vi "Test Recieved File Generation When Test Fails.vi"(11 "Test Case In":refnum<class "Basic Mechanics Tests.lvclass">) -> (0 "error out":errorcluster, 3 "Test Case Out":refnum<class "Basic Mechanics Tests.lvclass">)   [LabVIEW 2020, in "Basic Mechanics Tests.lvclass"]
uses:
  Basic Mechanics Tests.lvclass
  C:/Program Files/National Instruments/LabVIEW 2025/vi.lib/Astemes/LUnit/Test Case.lvclass
  Source/Approval Tests/Options/Options.lvclass
  Source/Approval Tests/Report Nothing/Report Nothing.lvclass
  C:/Users/SAS/Desktop/ApprovalTests.LabVIEW/Source/Approval Tests/Reporter/Reporter.lvclass
  Source/Approval Tests/Options/Options.lvclass/Options.ctl
  Source/Approval Tests/Naming Data/Naming Data.lvclass/Naming Data.ctl
  <vilib>/Astemes/LUnit/Test Case.lvclass/Test Case.ctl
  Source/Approval Tests/Scrubber/Scrubber.lvclass
  Source/Approval Tests/Namer/Namer.lvclass
  Source/Approval Tests/Naming Data/Naming Data.lvclass
  Source/Approval Tests/Reporter/Reporter.lvclass
  Source/Approval Tests/Text Comparator/Text Comparator.lvclass
  Basic Mechanics Tests.lvclass/Basic Mechanics Tests.ctl
  4be351cf-9afa-44a9-9686-c31d6937e1da.vi
  <vilib>/Astemes/LUnit/Test Case.lvclass
  5b6af433-73f2-478c-ac60-49e9a84e5db2.vi
  fbf3a6f1-25d3-4b1a-9ed1-fe282719be7b.vi
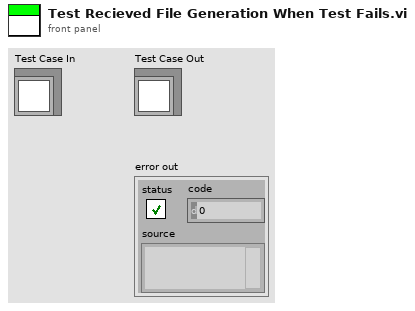
[diagram p1: front panel]
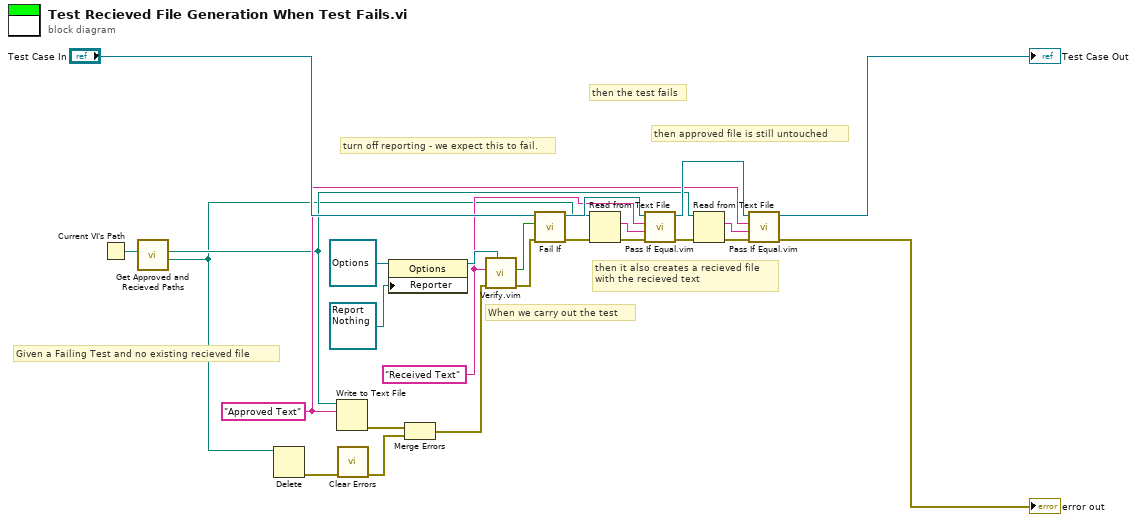
[diagram p0: block diagram]
diagram:
  w5 = "Approved Text"
  w9 = "Received Text"
  # "then approved file is still untouched"
  # "then it also creates a recieved file\nwith the recieved text"
  # "then the test fails"
  # "When we carry out the test"
  # "Given a Failing Test and no existing recieved file"
  # "turn off reporting - we expect this to fail."
  n1 = Current VI's Path() -> (path=w3:path)
  n2 = call "Get Approved and Recieved Paths.vi"("This VI"=w3) -> ("Recieved"=w1:path, "Approved Path"=w2:path)  [unwired: 9 in]
  n3 = Delete(path (use dialog)=w1) -> (error out=w25:errorcluster)  [unwired: 4 in, 2 out]
  n4 = Write to Text File(file (use dialog)=w2, text=w5) -> (error out=w24:errorcluster)  [unwired: 2 in, 2 out]
  n5 = call <vilib>:"Clear Errors.vi"("error in (no error)"=w25) -> ("error out"=w23:errorcluster)  [unwired: 5 in, 1 out]
  n6 = property on="Property Node" class="Options"(reference=refnum<class "Options.lvclass"> refnum ("Options"), "Reporter"=refnum<class "Report Nothing.lvclass"> refnum ("Approval Tests.lvlib:Report Nothing")) -> (reference out=w13:refnum<class "Options.lvclass">)  [unwired: 1 in, 1 out]
  n7 = Merge Errors(w24, w23) -> (w22:errorcluster)
  n8 = call "Verify.vim"("Options"=w13, "error in"=w22, "Anything"=w9) -> ("error out"=w18:errorcluster, "Passed?"=w11:bool)  [unwired: 6 in, 1 out]
  n9 = call <vilib>:"Fail If.vi"("error in (no error)"=w18, "Fail?"=w11, "LUnit Test Case In"="Test Case In") -> ("error out"=w17:errorcluster, "LUnit Test Case Out"=w10:refnum<class "Basic Mechanics Tests.lvclass">)  [unwired: 7 in]
  n10 = Read from Text File(file (use dialog)=w1, error in=w17) -> (text=w8:string, error out=w16:errorcluster)  [unwired: 2 in, 2 out]
  n11 = call "Pass If Equal.vim"("error in (no error)"=w16, "Actual"=w8, "Expected"=w9, "LUnit Test Case In"=w10) -> ("error out"=w19:errorcluster, "LUnit Test Case Out"=w7:refnum<class "Basic Mechanics Tests.lvclass">)  [unwired: 6 in]
  n12 = Read from Text File(file (use dialog)=w2, error in=w19) -> (text=w4:string, error out=w20:errorcluster)  [unwired: 2 in, 2 out]
  n13 = call "Pass If Equal.vim"("error in (no error)"=w20, "Actual"=w4, "Expected"=w5, "LUnit Test Case In"=w7) -> ("error out"=→"error out":errorcluster, "LUnit Test Case Out"=→"Test Case Out":refnum<class "Basic Mechanics Tests.lvclass">)  [unwired: 6 in]
